vi "按列提取EXCEL数据.vi"() -> ()   [LabVIEW 2014]
uses:
  <vilib>/Utility/file.llb/Read From Spreadsheet File (DBL).vi
panel:
  out "数据":dbl[](array[numeric])
  in  "file path (dialog if empty)":path caption="待提取文件路径"
  in  "停止":bool
  out "波形图":dbl[](graph)
  in  "查看第几列":u16(ring) items=["第1列", "第2列", "第3列", "第4列", "第5列", "第6列", "第7列", "第8列", "第9列", "第10列", "第11列", "第12列", "第13列", "第14列", "第15列", "第16列", "第17列", "第18列", "第19列", "第20列", "第21列", "第22列", "第23列", "第24列", "第25列", "第26列", "第27列", "第28列", "第29列", "第30列", "第31列", "第32列", "第33列", "第34列", "第35列", "第36列", "第37列", "第38列", "第39列", "第40列", "第41列", "第42列", "第43列", "第44列", "第45列", "第46列", "第47列", "第48列", "第49列", "第50列", "第51列", "第52列", "第53列", "第54列", "第55列", "第56列", "第57列"]
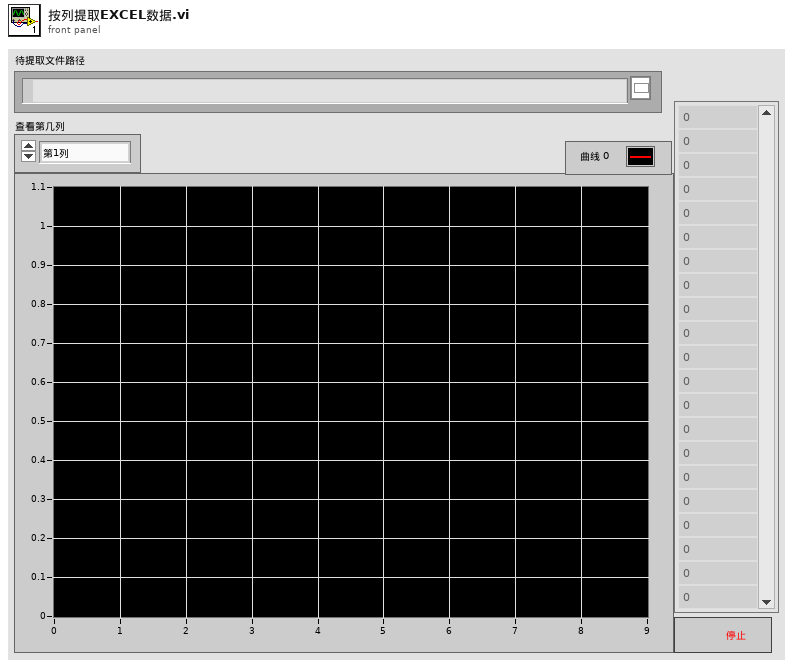
[diagram p1: front panel]
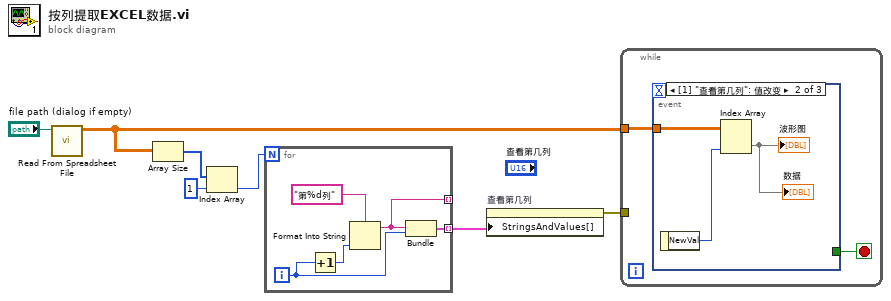
[diagram p0: block diagram]
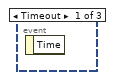
[diagram p2: hidden frame]
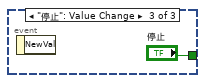
[diagram p3: hidden frame]
diagram:
  n1 = call-poly <vilib>:"Read From Spreadsheet File.vi"("file path (dialog if empty)"="file path (dialog if empty)") -> ("all rows"=w4:dbl[][])  [unwired: 6 in, 4 out]
  n2 = Array Size(array=w4) -> (size(s)=w7:i32[])
  n3 = Index Array(array=w7, index=1 ("索引")) -> (element=w5:i32)
  n4 = for {
    N: w5 -> [_]
    tunnel: [w9] -> w1 mode=indexing
    tunnel: [w8] -> _ mode=indexing
    i -> [w10]
    n5 = Increment(x=w10) -> (x+1=w12:i32)
    n6 = Format Into String(format string="第%d列" ("格式字符串"), w12) -> (resulting string=w8:string)  [unwired: 2 in, 1 out]
    n7 = Bundle(w8, w10) -> (w9:cluster{string, i32})  [unwired: 1 in]
  }
  n8 = property on="查看第几列" class="Ring (严格)"("StringsAndValues[]"=w1) -> (error out=w2:errorcluster)  [unwired: 2 in, 1 out]
  n9 = while {
    tunnel: w2 -> [_]
    tunnel: w4 -> [w14]
    stop <- w13 stop-if-true
    n10 = event shown="[1] \"查看第几列\": 值改变" {
      selector: _ -> [_ _ _]
      dyn-events: _ -> [_ _ _]
      timeout: _ -> [_ _ _]
      tunnel: w14 -> [_ w17 _]
      tunnel: [_ _ "停止"] -> w13
      event Timeout {
        n11 = event-data() -> ()  [unwired: 1 in, 1 out]
      }
      event "查看第几列": Value Change {
        n12 = event-data() -> ("NewVal"=w16:u16)  [unwired: 1 in]
        n13 = Index Array(array=w17, index (col)=w16) -> (element=→"波形图" →"数据":dbl[])  [unwired: 1 in]
      }
      event "停止": Value Change {
        n14 = event-data() -> ()  [unwired: 1 in, 1 out]
      }
    }
  }
